vi "3-2.vi"() -> ()   [LabVIEW 2022 SP3]
panel:
  out "波形图":cluster{i32, i32, dbl[]}[](graph)
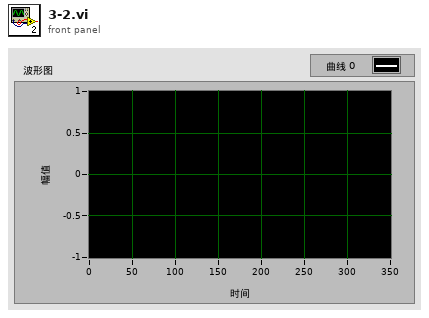
[diagram p1: front panel]
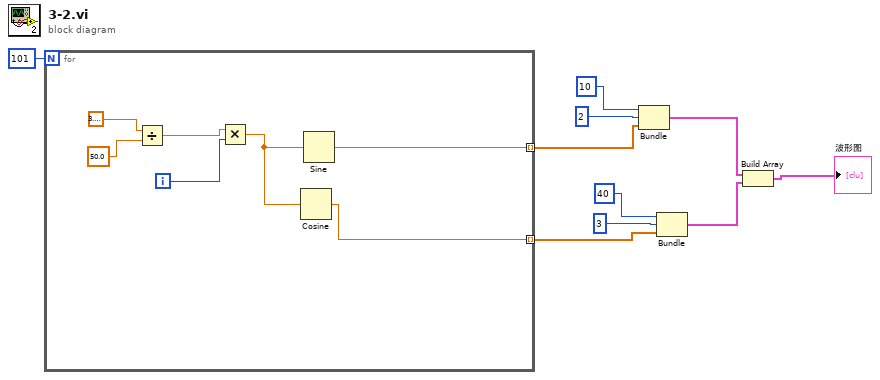
[diagram p0: block diagram]
diagram:
  n1 = for {
    N: 101 -> [_]
    tunnel: [w12] -> w7 mode=indexing
    tunnel: [w11] -> w4 mode=indexing
    i -> [w14]
    n2 = Divide(x=3.141592653589793, y=50.0) -> (x/y=w15:dbl)
    n3 = Multiply(x=w15, y=w14) -> (x*y=w13:dbl)
    n4 = Cosine(x=w13) -> (cos(x)=w11:dbl)
    n5 = Sine(x=w13) -> (sin(x)=w12:dbl)
  }
  n6 = Bundle(10, 2, w7) -> (w3:cluster{i32, i32, dbl[]})  [unwired: 1 in]
  n7 = Bundle(40, 3, w4) -> (w2:cluster{i32, i32, dbl[]})  [unwired: 1 in]
  n8 = Build Array(w3, w2) -> (→"波形图":cluster{i32, i32, dbl[]}[])
